vi "BfrPkt - Set Buffer Size Channel Value.vi"(8 "error in (no error)":errorcluster, 10 "Buffer Size":u32, 11 "Node Ptr":T1 format="%.0x") -> (0 "error out":errorcluster, 3 "Node Ptr out":T1 format="%.0x")   [LabVIEW 2019, in "UDP-Custom-Device System Explorer.lvlib"]
uses:
  UDP-Custom-Device System Explorer.lvlib
  <vilib>/NI VeriStand/Custom Device API/Custom Device Item Ref.ctl
  <vilib>/NI VeriStand/Custom Device Tools/Custom Device Utility Library/Custom Device Utility Library.lvlib
  <vilib>/NI VeriStand/Custom Device API/Custom Device API.lvlib
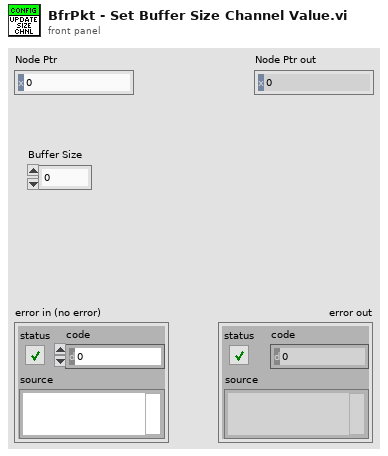
[diagram p1: front panel]
types:
  T1 = typedef "Custom Device API.lvlib/Custom Device Item Ref.ctl" = u64
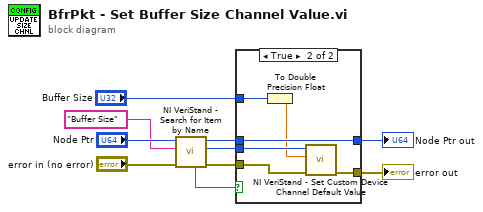
[diagram p0: block diagram]
diagram:
  n1 = call <vilib>:"NI VeriStand - Search for Item by Name.vi"("error in"="error in (no error)", "Item Name"="Buffer Size" ("Channel Name"), "Section Ref in"="Node Ptr") -> ("error out"=w6:errorcluster, "Item Ref"=w8:T1, "Section Ref out"=w3:T1, "Found"=w4:bool)  [unwired: 5 in]
  n2 = case shown="True" w4 {
    tunnel: w8 -> [_ w18]
    tunnel: [w12 w17] -> w7
    tunnel: w6 -> [w12 w16]
    tunnel: w3 -> [w11 w15]
    tunnel: [w11 w15] -> w2
    tunnel: "Buffer Size" -> [_ w14]
    frame False {
    }
    frame True {
      n3 = To Double Precision Float(number=w14) -> (double precision float=w13:dbl)
      n4 = call <vilib>:"NI VeriStand - Set Custom Device Channel Default Value.vi"("error in (no error)"=w16, "Default Value"=w13, "Channel Ref in"=w18) -> ("error out"=w17:errorcluster)  [unwired: 7 in, 1 out]
    }
  }
  "error out" <- w7
  "Node Ptr out" <- w2
